vi "Get RPI.SenseHat.Joystick.vi"(8 "error in (no error)":errorcluster, 11 "SenseHat in":refnum<class "SenseHat.lvclass">) -> (0 "error out":errorcluster, 2 "RPI.SenseHat.Joystick":refnum<class "RPI.SenseHat.Joystick.lvclass">, 3 "SenseHat out":refnum<class "SenseHat.lvclass">)   [LabVIEW 2020, in "RPI.SenseHat.lvlib" / "SenseHat.lvclass"]
uses:
  SenseHat.lvclass
  RPI.SenseHat.Joystick/Classes/senseHatJoystick/RPI.SenseHat.Joystick.lvclass
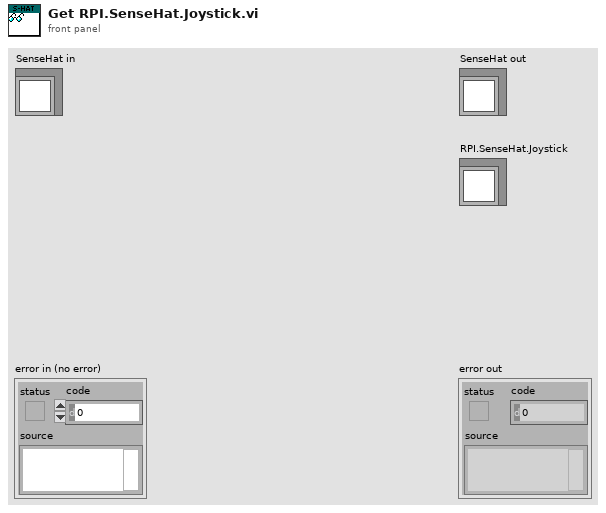
[diagram p1: front panel]
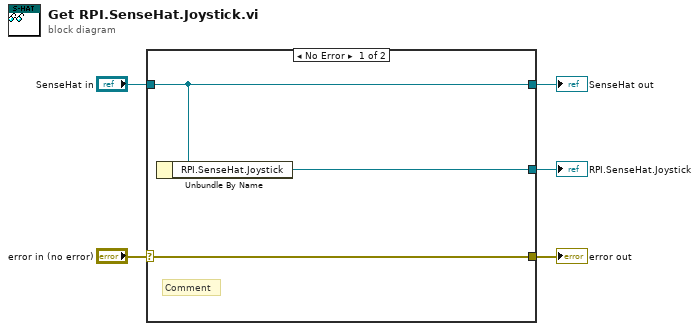
[diagram p0: block diagram]
diagram:
  n1 = case shown="No Error" "error in (no error)" {
    selector: "error in (no error)" -> [w8 w9]
    tunnel: [w8 w9] -> w4
    tunnel: [w7 w10] -> w2
    tunnel: "SenseHat in" -> [w7 w10]
    tunnel: [w6 _] -> w1
    frame No Error {
      # "Comment"
      n2 = Unbundle By Name(w7) -> ("RPI.SenseHat.Joystick"=w6:refnum<class "RPI.SenseHat.Joystick.lvclass">)
    }
    frame Error {
    }
  }
  "error out" <- w4
  "SenseHat out" <- w2
  "RPI.SenseHat.Joystick" <- w1
